vi "DamnYankeePWMCounter.vi"(6 "Jumped Up In":bool, 8 "Old Value":bool, 9 "New Value":bool, 10 "Counter In":i16, 11 "High Counter In":i16) -> (0 "Jumped Down Out":bool, 1 "Jumped Up Out":bool, 2 "Counter Out":i16, 3 "High Counter Out":i16, 4 "Ratio":sgl)   [LabVIEW 2013]
doc: "This VI looks for edges and counts both the number of steps it stays high and the total number of steps per cycle. It also indicates if the data stepped high or low.\n\nEric Schneider, May 2014"
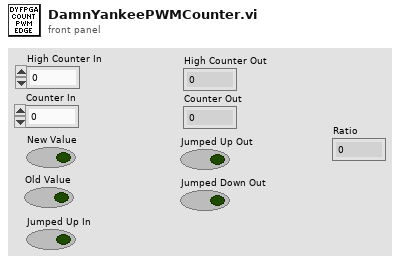
[diagram p1: front panel]
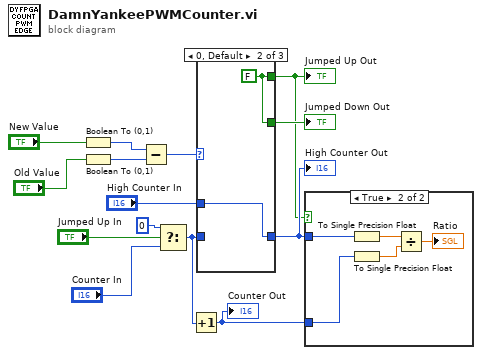
[diagram p0: block diagram]
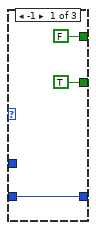
[diagram p3: hidden frame]
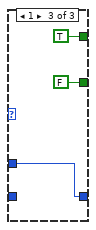
[diagram p4: hidden frame]
diagram:
  n1 = Boolean To (0,1)(Boolean="New Value") -> (0, 1=w12:i16)
  n2 = Boolean To (0,1)(Boolean="Old Value") -> (0, 1=w11:i16)
  n3 = Subtract(x=w12, y=w11) -> (x-y=w10:i16)
  n4 = Select(t=i16 0, s="Jumped Up In", f="Counter In") -> (s? t:f=w4:i16)
  n5 = Increment(x=w4) -> (x+1=w2:i16)
  "Counter Out" <- w2
  n6 = case shown="0, Default" w10 {
    tunnel: [FALSE ("Jumped Up") w18 TRUE ("Jumped Up In")] -> w1
    tunnel: w4 -> [w16 _ _]
    tunnel: [w16 w19 w22] -> w3
    tunnel: "High Counter In" -> [_ w19 w22]
    tunnel: [TRUE ("Jumped Up In") w18 FALSE ("Jumped Up In")] -> w8
    frame -1 {
    }
    frame 0, Default {
      w18 = FALSE ("Jumped Up In")
    }
    frame 1 {
    }
  }
  "Jumped Up Out" <- w1
  "High Counter Out" <- w3
  "Jumped Down Out" <- w8
  n7 = case shown="True" w1 {
    tunnel: w3 -> [_ w27]
    tunnel: w2 -> [_ w26]
    frame False {
    }
    frame True {
      n8 = To Single Precision Float(number=w27) -> (single precision float=w25:sgl)
      n9 = To Single Precision Float(number=w26) -> (single precision float=w24:sgl)
      n10 = Divide(x=w25, y=w24) -> (x/y=→"Ratio":sgl)
    }
  }
